vi "TAT-ASS-Alarm Display.vi"(11 "Ass Alarm":u16[](array[numeric])) -> ()   [LabVIEW 2017]
panel:
  in  "stop":bool
  out "Alarm List":string
  # "ASS ALARMS"
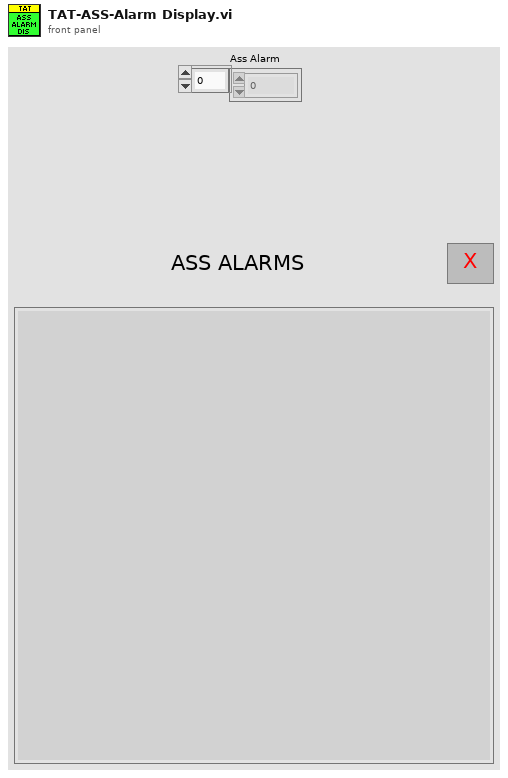
[diagram p1: front panel]
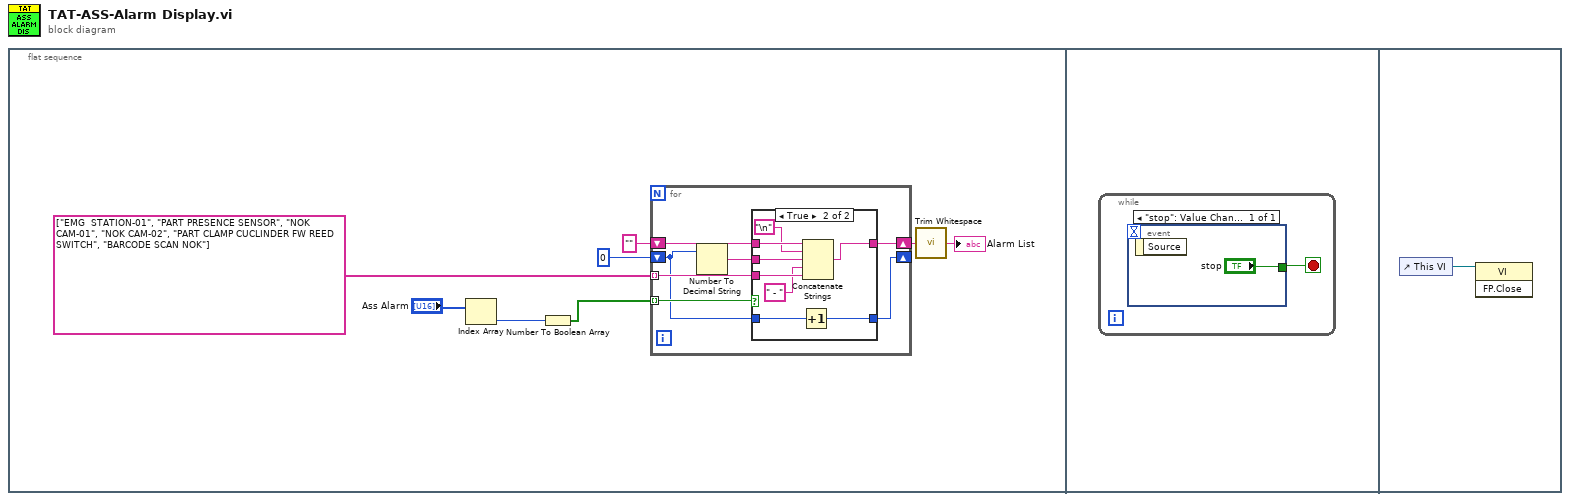
[diagram p0: block diagram]
diagram:
  n1 = flat-sequence {
    frame #0 {
      n2 = Index Array(array="Ass Alarm") -> (element=w1:u16)  [unwired: 1 in]
      n3 = Number To Boolean Array(number=w1) -> (Boolean array=w2:bool[])
      n4 = for {
        tunnel: w2 -> [w14] mode=indexing
        tunnel: string[] ["EMG  STATION-01", "PART PRESENCE SENSOR", "NOK CAM-01", "NOK CAM-02", "PART CLAMP CUCLINDER FW REED SWITCH", "BARCODE SCAN NOK"] -> [w12] mode=indexing
        shift-right: [w13] -> w6
        shift-left: "" -> [w15]
        shift-right: [w10] -> _
        shift-left: u8 0 -> [w9]
        n5 = Number To Decimal String(number=w9) -> (decimal integer string=w11:string)  [unwired: 1 in]
        n6 = case shown="True" w14 {
          tunnel: w15 -> [w17 w25]
          tunnel: [w17 w23] -> w13
          tunnel: w12 -> [_ w21]
          tunnel: w11 -> [_ w22]
          tunnel: [w16 w18] -> w10
          tunnel: w9 -> [w16 w19]
          frame False {
          }
          frame True {
            n7 = Increment(x=w19) -> (x+1=w18:u8)
            n8 = Concatenate Strings(w25, "\n", w22, " - ", w21) -> (w23:string)
          }
        }
      }
      n9 = call <vilib>:"Trim Whitespace.vi"("string"=w6) -> ("trimmed string"=→"Alarm List":string)  [unwired: 1 in]
    }
    frame #1 {
      n10 = while {
        stop <- w26 stop-if-true
        n11 = event shown="[0] \"stop\": Value Change" {
          selector: _ -> [_]
          dyn-events: _ -> [_]
          timeout: _ -> [_]
          tunnel: ["stop"] -> w26
          event "stop": Value Change {
            n12 = event-data() -> ()  [unwired: 1 in, 1 out]
          }
        }
      }
    }
    frame #2 {
      n13 = control-ref of="This VI"() -> (w28:refnum<vi>)
      n14 = invoke class="VI" method="FP.Close"(reference=w28) -> ()  [unwired: 2 in, 3 out]
    }
  }
